vi "Main UI.vi"(8 "error in (no error)":errorcluster, 11 "SOL-Server in":refnum<class "SOL-Server.lvclass">) -> (0 "error out":errorcluster, 3 "SOL-Server out":refnum<class "SOL-Server.lvclass">)   [LabVIEW 2020, in "Summer of LabVIEW.lvlib" / "SOL-Server.lvclass"]
uses:
  SOL-Server.lvclass
  <vilib>/IlluminatedG/IG HTTP Server/HTTP Server/Trace Log.ctl
  <vilib>/IlluminatedG/IG HTTP Server/HTTP Server/Trace Item.ctl
  <vilib>/IlluminatedG/IG HTTP Server/HTTP Server/Processing Step.ctl
  <vilib>/IlluminatedG/IG HTTP Utils/HTTP Utils/Method.ctl
  Error Log.ctl
  UI State.ctl
  SOL-Server.lvclass/SOL-Server.ctl
  <vilib>/IlluminatedG/IG HTTP Server/HTTP Server/Server/Server.lvclass
  <vilib>/IlluminatedG/IG HTTP Server/HTTP Server/RequestTraceLog/RequestTraceLog.lvclass
  SOL-Config/SOL-Config.lvclass
  Challenge DB/Challenge DB.lvclass
  Leaderboard/Leaderboard.lvclass
  <vilib>/IlluminatedG/IG HTTP Server/HTTP Server/HTTP Server.lvlib
  <vilib>/IlluminatedG/IG HTTP Utils/HTTP Utils/HTTP Utils.lvlib
panel:
  in  "Tabs":enum32{"Traces", "Errors", "Config"}(tab)
  out "Trace Logs":T1[](array[typedef]) {"Sending" format="%_6f"; "Expires" format="%<%X %x>T"; "Created" format="%<%X %x>T"; "Waiting" format="%_6f"; "Parsing" format="%_6f"; "Processing" format="%_6f"; "Items"."Time" format="%.6f"; "Items"."Duration" format="%.6f"}
  in  "Traces":bool
  in  "Errors":bool
  in  "Limit":i32=10000
  out "Errors":T5[](array[typedef])
  in  "Active Chal ID":i64
  # "Request"
  # "Response"
  # "Session"
  # "Auth"
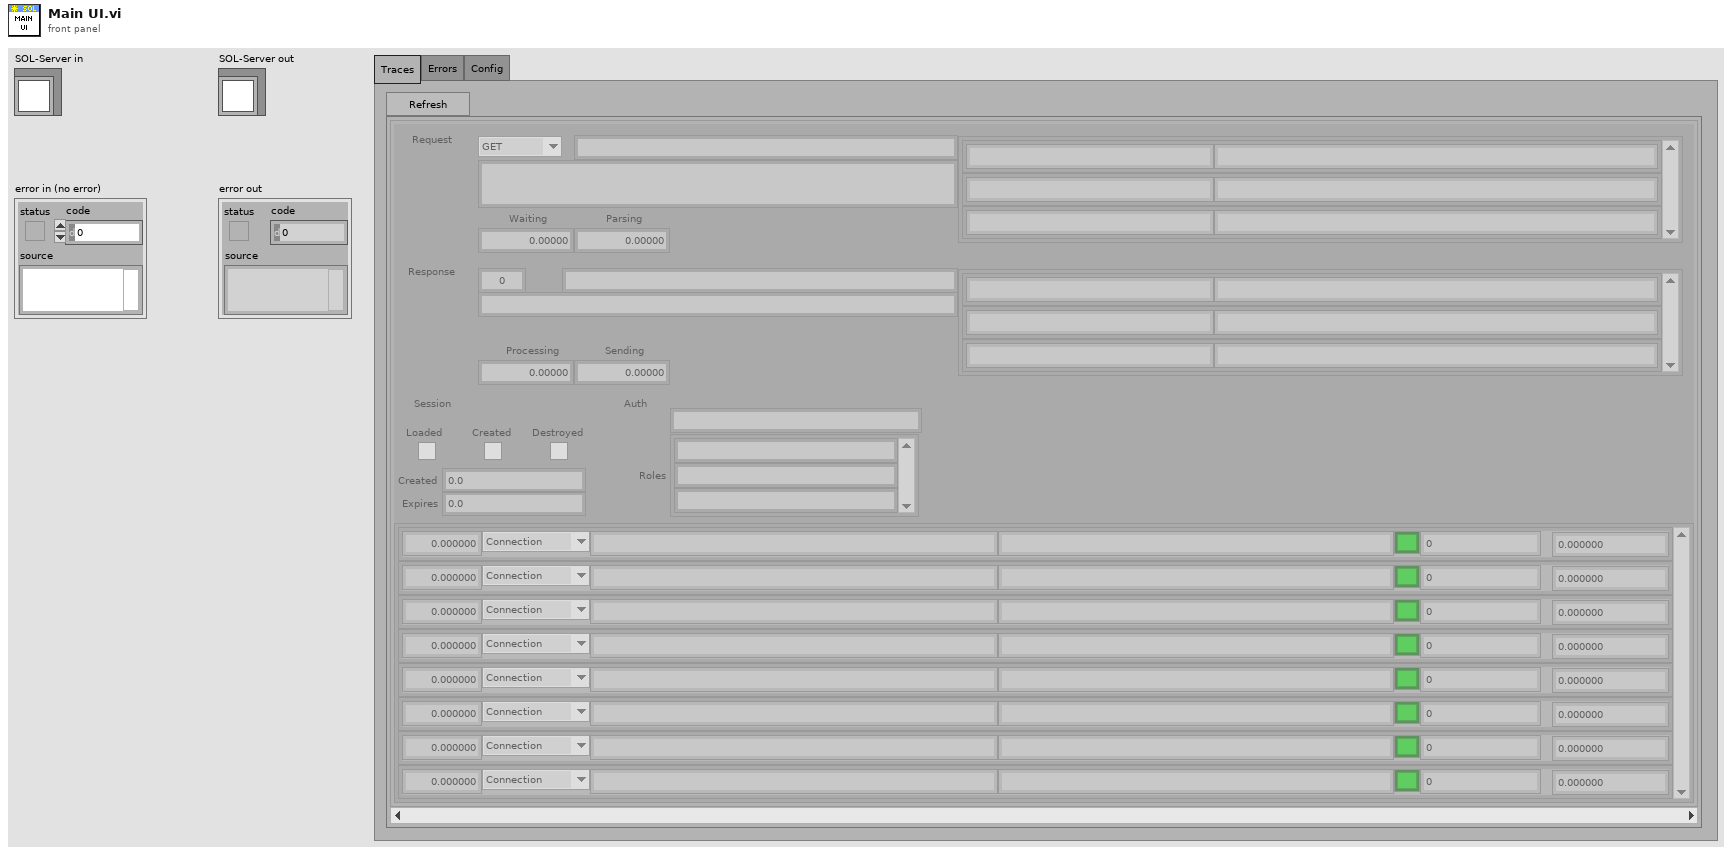
[diagram p1: front panel]
types:
  T1 = typedef "HTTP Server.lvlib/Trace Log.ctl" = cluster{"Items":T2[], "Client":string, "Target":string, "Response Type":string, "Processing":dbl, "Status":u16, "Method":T4, "Content Type":string, "Request Headers":cluster{"Name":string, "Value":string}[], "Parsing":dbl, "Waiting":dbl, "Identity":string, "Loaded":bool, "Created":bool, "Destroyed":bool, "Response Headers":cluster{"Name":string, "Value":string}[], "Created":dbl, "Expires":dbl, "Roles":string[], "Sending":dbl}
  T2 = typedef "HTTP Server.lvlib/Trace Item.ctl" = cluster{"Duration":dbl, "Step":T3, "Class":string, "Info":string, "Status":bool, "Code":i32, "Time":dbl}
  T3 = typedef "HTTP Server.lvlib/Processing Step.ctl" = enum16{"Connection", "Request", "Routing", "Controller Init", "Controller", "Response", "Complete", "Exception"}
  T4 = typedef "HTTP Utils.lvlib/Method.ctl" = enum16{"GET", "HEAD", "POST", "PUT", "DELETE", "CONNECT", "OPTIONS", "TRACE", "PATCH"}
  T5 = typedef "Summer of LabVIEW.lvlib/SOL-Server.lvclass/Error Log.ctl" = cluster{"Time Stamp":timestamp, "Code":i32, "Source":string}
  T6 = typedef "Summer of LabVIEW.lvlib/SOL-Server.lvclass/UI State.ctl" = enum16{"Init", "Run", "Close"}
  T7 = enum32{"Invalid", "Standard", "Closed", "Hidden", "Minimized", "Maximized"}
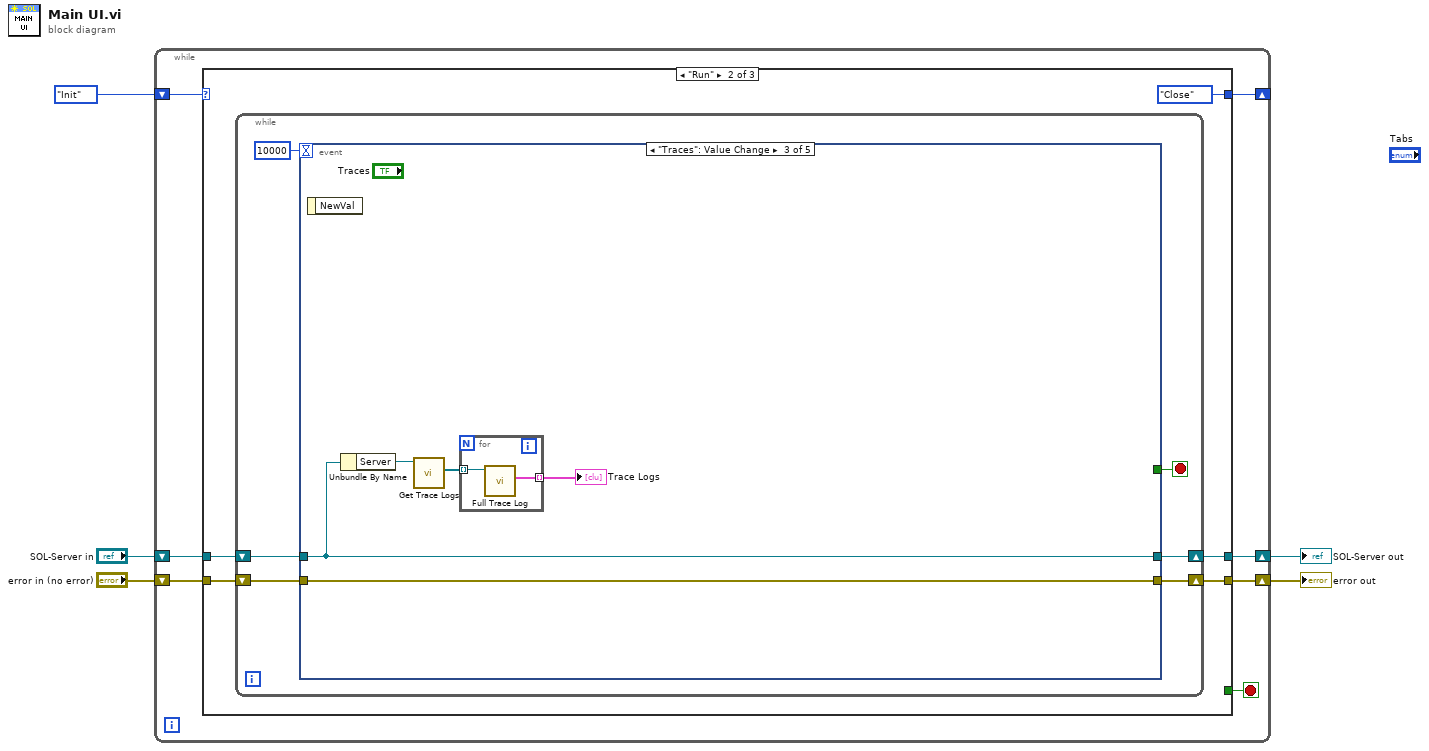
[diagram p0: block diagram]
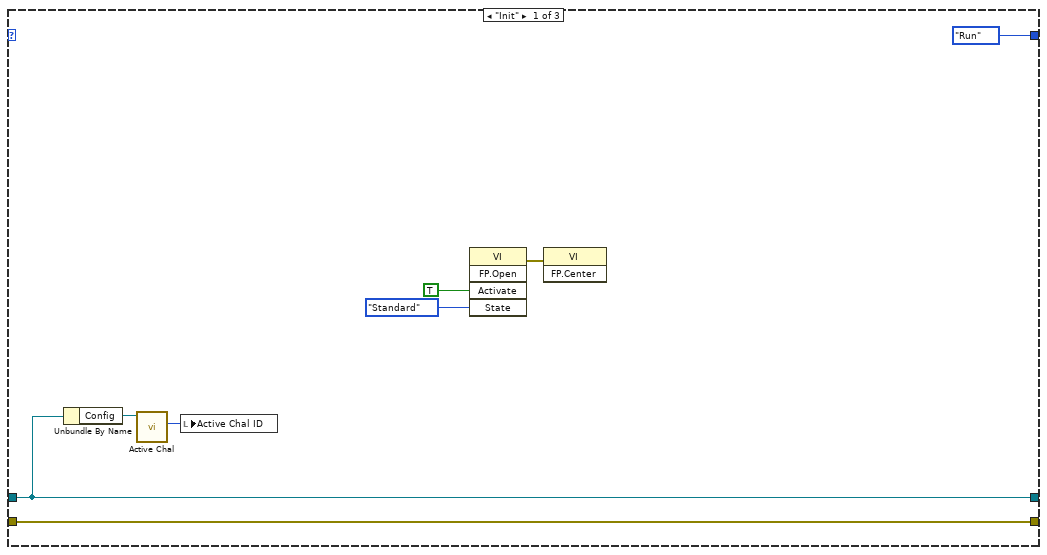
[diagram p2: hidden frame]
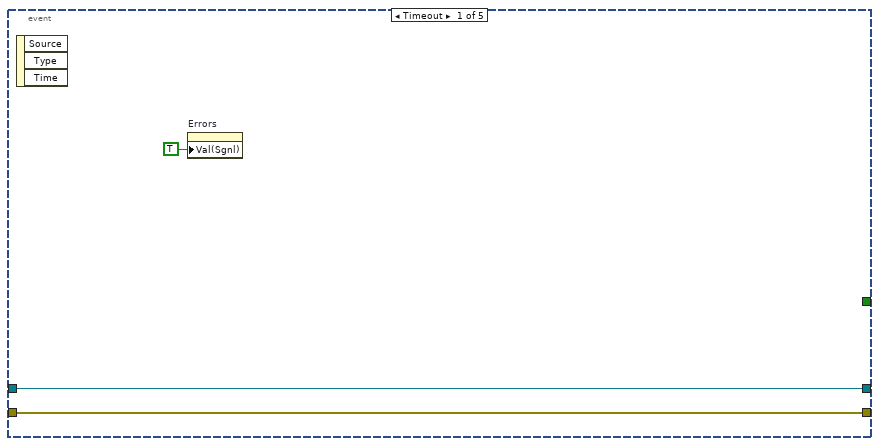
[diagram p3: hidden frame]
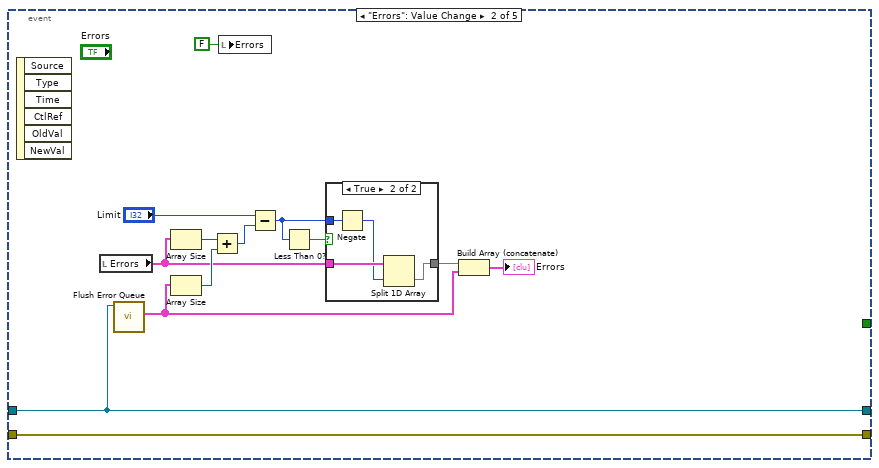
[diagram p4: hidden frame]
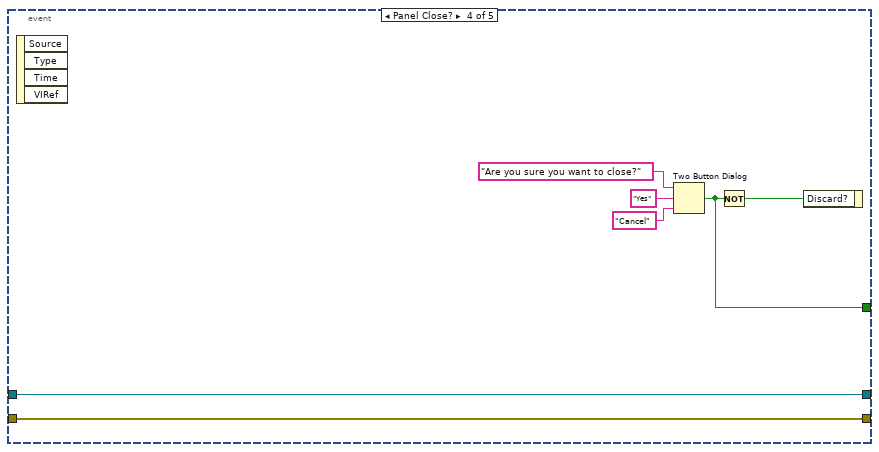
[diagram p6: hidden frame]
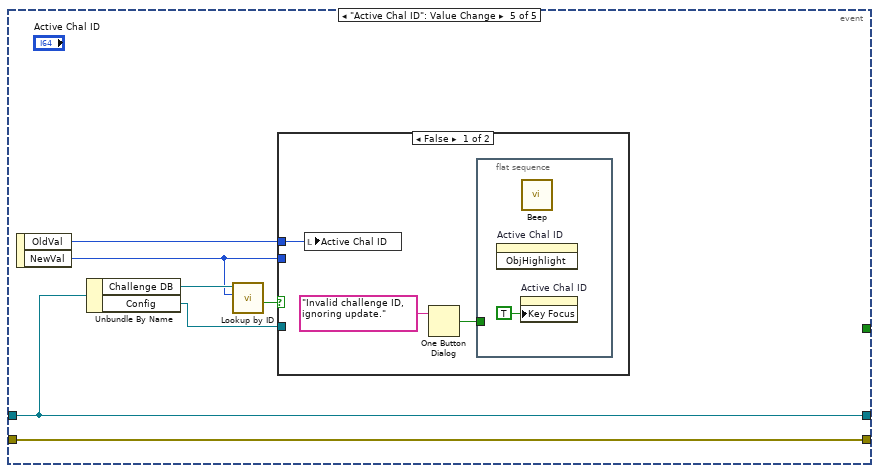
[diagram p7: hidden frame]
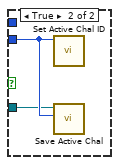
[diagram p8: hidden frame]
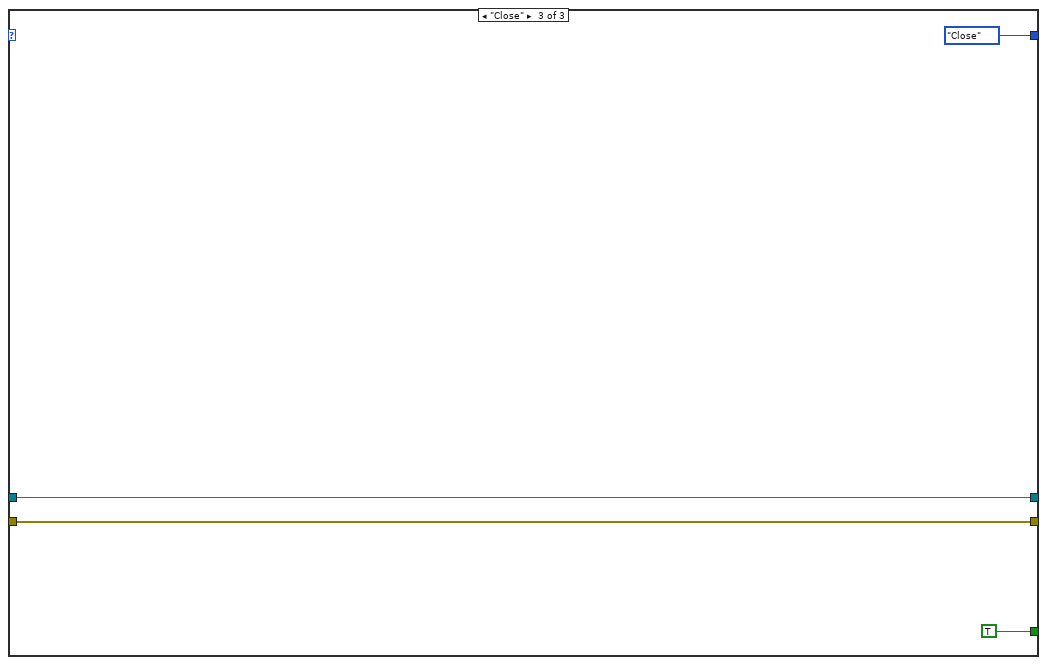
[diagram p9: hidden frame]
diagram:
  n1 = while {
    shift-right: [w8] -> w4
    shift-left: "SOL-Server in" -> [w10]
    shift-right: [w7] -> w2
    shift-left: "error in (no error)" -> [w9]
    shift-right: [w11] -> _
    shift-left: UI_State."Init" ("UI State") -> [w12]
    stop <- w6 stop-if-true
    n2 = case shown="\"Run\"" w12 {
      tunnel: [UI_State."Run" ("UI State") UI_State."Close" ("UI State") UI_State."Close" ("UI State")] -> w11
      tunnel: w10 -> [w15 w24 w82]
      tunnel: w9 -> [w19 w23 w81]
      tunnel: [w15 w22 w82] -> w8
      tunnel: [w19 w21 w81] -> w7
      tunnel: [_ _ TRUE] -> w6
      frame "Init" {
        n3 = Unbundle By Name(w15) -> ("Config"=w14:refnum<class "SOL-Config.lvclass">)
        n4 = call "Active Chal.vi"("SOL-Config in"=w14) -> ("Active Chal"=w13:i64)  [unwired: 8 in, 2 out]
        n5 = local write "Active Chal ID"(w13) -> ()
        n6 = invoke class="VI" method="FP.Open"("Activate"=TRUE ("Activate?"), "State"=T7."Standard") -> (error out=w16:errorcluster)  [unwired: 3 in, 4 out]
        n7 = invoke class="VI" method="FP.Center"(error in=w16) -> ()  [unwired: 2 in, 3 out]
      }
      frame "Run" {
        n8 = while {
          shift-right: [w29] -> w22
          shift-left: w24 -> [w31]
          shift-right: [w28] -> w21
          shift-left: w23 -> [w30]
          stop <- w27 stop-if-true
          n9 = event shown="[2] \"Traces\": Value Change" {
            selector: _ -> [_ _ _ _ _]
            dyn-events: _ -> [_ _ _ _ _]
            timeout: 10000 -> [_ _ _ _ _]
            tunnel: w31 -> [w33 w35 w56 w66 w72]
            tunnel: w30 -> [w34 w47 w57 w65 w73]
            tunnel: [w33 w35 w56 w66 w72] -> w29
            tunnel: [w34 w47 w57 w65 w73] -> w28
            tunnel: [_ _ _ w61 _] -> w27
            event Timeout {
              n10 = event-data() -> ()  [unwired: 1 in, 3 out]
              n11 = property on="Errors" class="Bool (strict)"("Val(Sgnl)"=TRUE ("Value (Signaling)")) -> ()  [unwired: 2 in, 2 out]
            }
            event "Errors": Value Change {
              n12 = event-data() -> ()  [unwired: 1 in, 6 out]
              n13 = local read "Errors"() -> (w39:T5[])
              n14 = call "Flush Error Queue.vi"("SOL-Server in"=w35) -> ("Errors"=w38:T5[])  [unwired: 8 in, 2 out]
              n15 = Array Size(array=w39) -> (size(s)=w45:i32)
              n16 = Array Size(array=w38) -> (size(s)=w44:i32)
              n17 = Add(x=w45, y=w44) -> (x+y=w43:i32)
              n18 = local write "Errors"(FALSE ("Errors")) -> ()
              n19 = Subtract(x="Limit", y=w43) -> (x-y=w40:i32)
              n20 = Less Than 0?(x=w40) -> (x < 0?=w41:bool)
              n21 = case shown="True" w41 {
                tunnel: w40 -> [_ w52]
                tunnel: w39 -> [w48 w51]
                tunnel: [w48 w49] -> w37
                frame False {
                }
                frame True {
                  n22 = Negate(x=w52) -> (-x=w50:i32)
                  n23 = Split 1D Array(array=w51, index=w50) -> (second subarray=w49:T5[])  [unwired: 1 out]
                }
              }
              n24 = Build Array (concatenate)(w37, w38) -> (→"Errors":T5[])
            }
            event "Traces": Value Change {
              n25 = event-data() -> ()  [unwired: 1 in, 1 out]
              n26 = Unbundle By Name(w56) -> ("Server"=w55:refnum<class "Server.lvclass">)
              n27 = call <vilib>:"Get Trace Logs.vi"("Server in"=w55) -> ("Trace Logs"=w54:refnum<class "RequestTraceLog.lvclass">[])  [unwired: 8 in, 2 out]
              n28 = for {
                tunnel: w54 -> [w59] mode=indexing
                tunnel: [w58] -> w53 mode=indexing
                n29 = call <vilib>:"Full Trace Log.vi"("RequestTraceLog in"=w59) -> ("Trace Log"=w58:T1)  [unwired: 8 in, 2 out]
              }
              "Trace Logs" <- w53
            }
            event Panel Close? {
              n30 = event-data() -> ()  [unwired: 1 in, 4 out]
              n31 = Two Button Dialog(message="Are you sure you want to close?", 1:"Cancel" ("T button name (\"OK\")"), 2:"Yes" ("T button name (\"OK\")")) -> (T button?=w61:bool)
              n32 = Not(x=w61) -> (.not. x?=w60:bool)
              n33 = event-data("Discard?"=w60) -> ()  [unwired: 1 in, 1 out]
            }
            event "Active Chal ID": Value Change {
              n34 = event-data() -> ("OldVal"=w67:i64, "NewVal"=w69:i64)  [unwired: 1 in]
              n35 = Unbundle By Name(w72) -> ("Challenge DB"=w71:refnum<class "Challenge DB.lvclass">, "Config"=w68:refnum<class "SOL-Config.lvclass">)
              n36 = call "Lookup by ID.vi"("ID"=w69, "Challenge DB in"=w71) -> ("Found?"=w70:bool)  [unwired: 6 in, 3 out]
              n37 = case shown="False" w70 {
                tunnel: w69 -> [_ w79]
                tunnel: w68 -> [_ w78]
                tunnel: w67 -> [w76 _]
                frame False {
                  n38 = local write "Active Chal ID"(w76) -> ()
                  n39 = One Button Dialog(message="Invalid challenge ID, ignoring update.") -> (true=w74:bool)  [unwired: 1 in]
                  n40 = flat-sequence {
                    tunnel: w74 -> [_]
                    frame #0 {
                      n41 = invoke on="Active Chal ID" class="DigNum (strict)" method="ObjHighlight"() -> ()  [unwired: 3 in, 3 out]
                      n42 = property on="Active Chal ID" class="DigNum (strict)"("Key Focus"=TRUE) -> ()  [unwired: 2 in, 2 out]
                      n43 = call <vilib>:"Beep.vi"() -> ()  [unwired: 12 in]
                    }
                  }
                }
                frame True {
                  n44 = call "Set Active Chal ID.vi"("Active Chal ID"=w79) -> ()  [unwired: 10 in, 1 out]
                  n45 = call "Save Active Chal.vi"("Active Chal"=w79, "SOL-Config in"=w78) -> ()  [unwired: 8 in, 2 out]
                }
              }
            }
          }
        }
      }
      frame "Close" {
      }
    }
  }
  "error out" <- w2
  "SOL-Server out" <- w4
